vi "Remove Pipe.vi"(8 "error in (no error)":errorcluster, 11 "pathname in":string) -> (0 "error out":errorcluster)   [LabVIEW 2013, in "Linux RT IPC.Pipes.lvlib"]
doc: "This VI removes the pipe from the filesystem. Exisiting endpoints currently using the pipe can continue to do so, but no new endpoints can be created once the pipe is removed."
uses:
  Linux RT IPC.Pipes.lvlib
  C/SubVIs/error handler.vi
  <vilib>/NI/NI Linux RT Errno/VIs/Public/Get Errno Value for Calling Thread.vi
  C/Linux RT IPC.C.lvlib
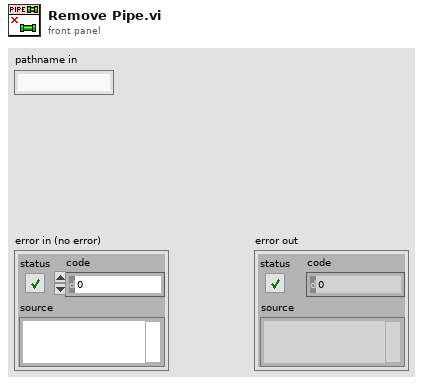
[diagram p1: front panel]
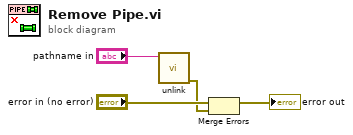
[diagram p0: block diagram]
diagram:
  n1 = call "unlink.vi"("pathname"="pathname in") -> ("error out"=w2:errorcluster)  [unwired: 10 in]
  n2 = Merge Errors("error in (no error)", w2) -> (→"error out":errorcluster)
